vi "pid.vi"(6 "y":dbl, 7 "setpoint":dbl format="%#_13g", 9 "kd":dbl, 11 "kp":dbl) -> (3 "Motor Command":dbl)   [LabVIEW 2015]
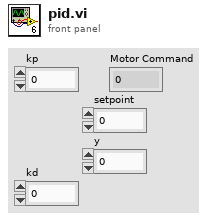
[diagram p1: front panel]
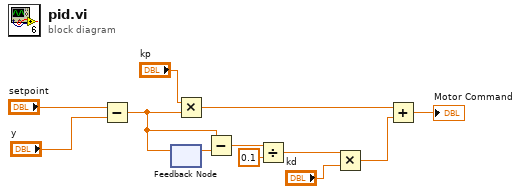
[diagram p0: block diagram]
diagram:
  n1 = Subtract(x="setpoint", y="y") -> (x-y=w6:dbl)
  n2 = feedback #1() -> (w5:dbl)  [unwired: 1 in]
  n3 = feedback-in #1(w6) -> ()
  n4 = Multiply(x="kp", y=w6) -> (x*y=w1:dbl)
  n5 = Subtract(x=w6, y=w5) -> (x-y=w7:dbl)
  n6 = Divide(x=w7, y=0.1) -> (x/y=w10:dbl)
  n7 = Multiply(x=w10, y="kd") -> (x*y=w11:dbl)
  n8 = Add(x=w1, y=w11) -> (x+y=→"Motor Command":dbl)
